vi "RSNRPZ Close.vi"(8 "error in (no error)":errorcluster, 11 "VISA session":refnum<visa-resource-name> caption="VISA resource name") -> (0 "error out":errorcluster)   [LabVIEW 2010]
doc: "This VI disconnect all channels and close driver session."
uses:
  rsnrpz_32.dll
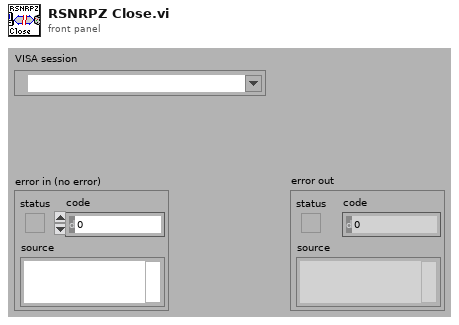
[diagram p1: front panel]
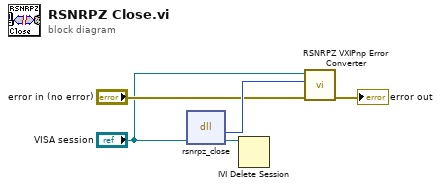
[diagram p0: block diagram]
diagram:
  n1 = dll-call lib="rsnrpz_32.DLL" fn="rsnrpz_close"("instrumentHandle"="VISA session") -> ("return type"=w4:i32)  [unwired: 4 in, 2 out]
  n2 = IVI Delete Session(11:"VISA session") -> ()
  n3 = call <instrlib>:"RSNRPZ VXIPnp Error Converter.vi"("error in"="error in (no error)", "VXIPnp error code"=w4, "VISA session"="VISA session") -> ("error out"=→"error out":errorcluster)  [unwired: 7 in, 1 out]
